vi "GetCustomDeviceXMLVIs.vi"(8 "error in (no error)":errorcluster, 11 "absolute custom device xml file":path) -> (0 "error out":errorcluster, 3 "custom device VIs":T1(array[cluster]))   [LabVIEW 2027, in "VeriStandTestUtilities.lvlib"]
uses:
  VeriStandTestUtilities.lvlib
  C:/NetCoreDLL/NationalInstruments.VeriStand.SystemStorage.dll
  NetCoreDLL/NationalInstruments.VeriStand.SystemStorage.dll
  C:/NetCoreDLL/NationalInstruments.VeriStand.XMLReader.dll
  NetCoreDLL/NationalInstruments.VeriStand.XMLReader.dll
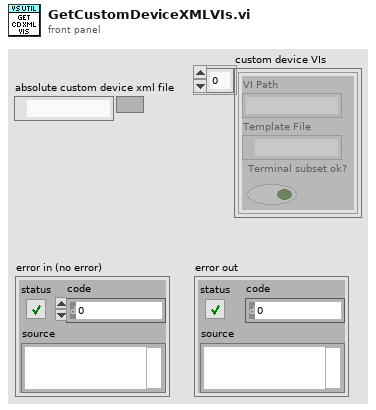
[diagram p1: front panel]
types:
  T1 = cluster{"VI Path":string, "Template File":path, "Terminal subset ok?":bool}[]
  T2 = cluster{"Item2Launch":refnum<k39>, "Template File":path, "Terminal subset ok?":bool}
  T3 = cluster{"Item2Launch":refnum<k39>, "Template File":path, "Terminal subset ok?":bool}[]
  T4 = cluster{"Source":refnum<k39>, "Folder Path":path, "Terminal subset ok?":bool}[]
  T5 = cluster{"Location":refnum<k39>, path, "Terminal subset ok?":bool}[]
  T6 = cluster{"Location":refnum<k39>, "Folder Path":path, "Terminal subset ok?":bool}[]
  T7 = cluster{"Path1":string, "appended path":path, "Terminal subset ok?":bool}[]
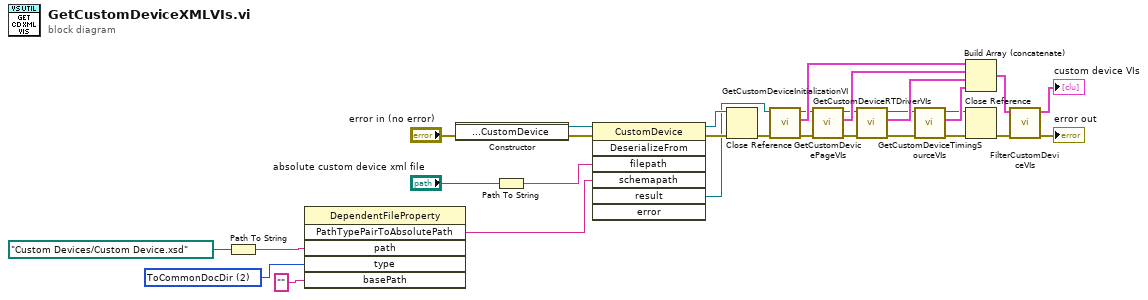
[diagram p0: block diagram]
diagram:
  w22 = 2 items=["Absolute", "Relative", "ToCommonDocDir", "ToApplicationDataDir"] ("type")
  n1 = Path To String(path=path "Custom Devices/Custom Device.xsd") -> (string=w24:string)
  n2 = invoke class="DependentFileProperty" method="PathTypePairToAbsolutePath"("path"=w24, "type"=w22, "basePath"="") -> ("PathTypePairToAbsolutePath"=w19:string)  [unwired: 3 in, 5 out]
  n3 = constructor class="CustomDevice"(error in="error in (no error)") -> (reference out=w28:refnum<k39>, error out=w29:errorcluster)  [unwired: 2 in, 1 out]
  n4 = Path To String(path="absolute custom device xml file") -> (string=w26:string)
  n5 = invoke class="CustomDevice" method="DeserializeFrom"(reference=w28, error in=w29, "filepath"=w26, "schemapath"=w19) -> (reference out=w20:refnum<k39>, error out=w21:errorcluster, "result"=w7:refnum<k39>)  [unwired: 3 in, 4 out]
  n6 = Close Reference(reference=w20, error in (no error)=w21) -> (error out=w5:errorcluster)
  n7 = call "GetCustomDeviceInitializationVI.vi"("error in (no error)"=w5, "NationalInstruments.VeriStand.CustomDevice.CustomDevice"=w7) -> ("error out"=w11:errorcluster, "initialization VI"=w16:T2, "NationalInstruments.VeriStand.CustomDevice.CustomDevice"=w10:refnum<k39>)  [unwired: 7 in]
  n8 = call "GetCustomDevicePageVIs.vi"("error in (no error)"=w11, "NationalInstruments.VeriStand.CustomDevice.CustomDevice"=w10) -> ("error out"=w12:errorcluster, "page VIs"=w15:T3, "NationalInstruments.VeriStand.CustomDevice.CustomDevice"=w9:refnum<k39>)  [unwired: 7 in]
  n9 = call "GetCustomDeviceRTDriverVIs.vi"("error in (no error)"=w12, "NationalInstruments.VeriStand.CustomDevice.CustomDevice"=w9) -> ("error out"=w4:errorcluster, "RT driver VIs"=w14:T4, "NationalInstruments.VeriStand.CustomDevice.CustomDevice"=w2:refnum<k39>)  [unwired: 7 in]
  n10 = call "GetCustomDeviceTimingSourceVIs.vi"("error in (no error)"=w4, "NationalInstruments.VeriStand.CustomDevice.CustomDevice"=w2) -> ("error out"=w3:errorcluster, "timing source VIs"=w6:T5, "NationalInstruments.VeriStand.CustomDevice.CustomDevice"=w1:refnum<k39>)  [unwired: 7 in]
  n11 = Build Array (concatenate)(w16, w15, w14, w6) -> (w13:T6)
  n12 = Close Reference(reference=w1, error in (no error)=w3) -> (error out=w8:errorcluster)
  n13 = call "FilterCustomDeviceVIs.vi"("error in (no error)"=w8, "custom device VIs in"=w13) -> ("error out"=→"error out":errorcluster, "custom device VIs out"=→"custom device VIs":T7)  [unwired: 8 in]
